vi "myRIO__TCP_disconnect_forWrite.vi"(8 "input_error":errorcluster, 11 "input_hTCP":refnum<k5>) -> (0 "output_error":errorcluster)   [LabVIEW 2014]
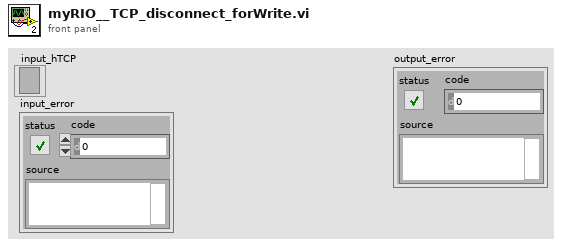
[diagram p1: front panel]
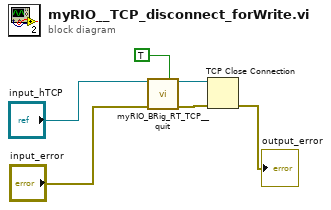
[diagram p0: block diagram]
diagram:
  n1 = call "myRIO_BRig_RT_TCP__quit.vi"("input_hTCP"="input_hTCP", "input_I_connected_TCP"=TRUE, "input_error"="input_error") -> ("output_hTCP"=w3:refnum<k5>, "output_error"=w2:errorcluster)  [unwired: 11 in]
  n2 = TCP Close Connection(connection ID=w3, error in (no error)=w2) -> (error out=→"output_error":errorcluster)  [unwired: 1 in, 1 out]
